vi "Main-Control Pannel.vi"() -> ()   [LabVIEW 2014]
panel:
  in  "Wifi Channel":i32=3
  out "ERROR":bool
  in  "remote IP Address":string="192.168.1.103"
  in  "UDP setup":T1={"remote IP Address"="127.0.0.0", "remote port"=54322, "local port(Tx)"=54321, "local port(Rx)"=54323}
  in  "USRP setup":T2={"Active Antenna"="RX2", "Carrier Frequency"=0.0, "IQ Rate"=0.0, "Gain"=0.0}
  in  "device names":refnum<k15>="192.168.10.2"
  in  "USRP input cluster":T3
  in  "UDP input cluster":T4
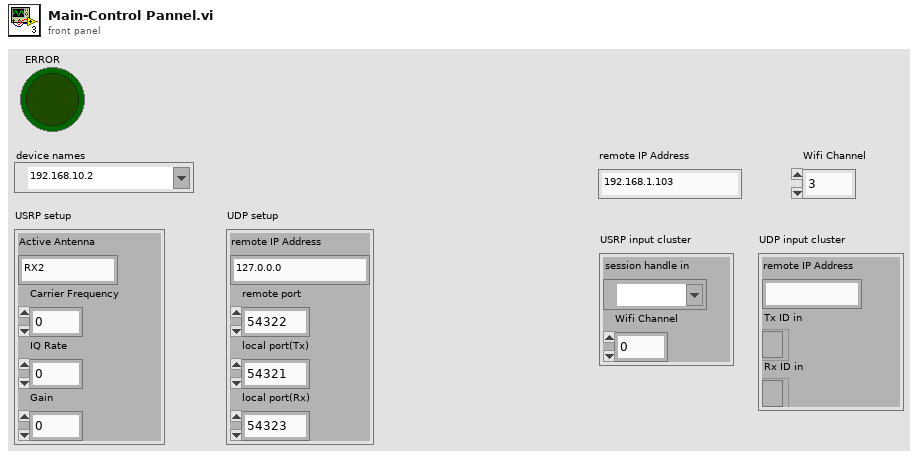
[diagram p1: front panel]
types:
  T1 = cluster{"remote IP Address":string, "remote port":u16, "local port(Tx)":u16, "local port(Rx)":u16}
  T2 = cluster{"Active Antenna":string, "Carrier Frequency":dbl, "IQ Rate":dbl, "Gain":dbl}
  T3 = cluster{"session handle in":refnum<k15>, "Wifi Channel":i32}
  T4 = cluster{"remote IP Address":string, "Tx ID in":refnum<k16>, "Rx ID in":refnum<k16>}
  T5 = cluster{"Tx ID out":refnum<k16>, "Rx ID out":refnum<k16>, "Delay Estimation":cluster{"next status(max)":i32, "next probability(max)":dbl}}
  T6 = cluster{"session handle out":refnum<k15>, "Power Estimation":cluster{"next status(max)":i32, "next probability(max)":dbl}}
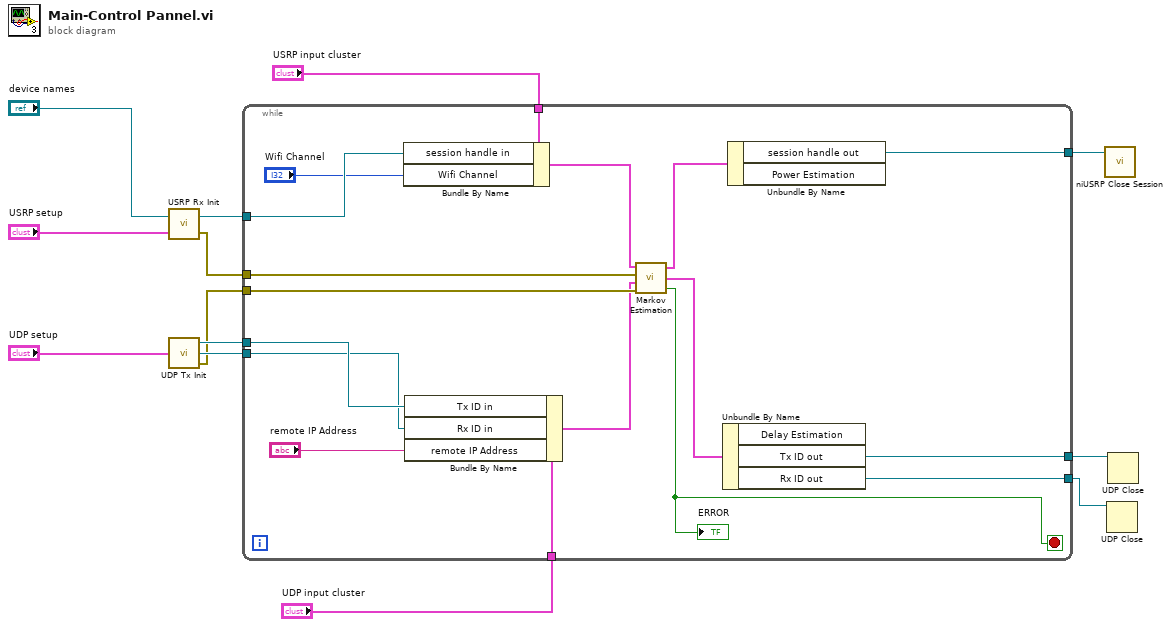
[diagram p0: block diagram]
diagram:
  n1 = call "USRP Rx Init.vi"("setup para"="USRP setup", "device names"="device names") -> ("error out"=w7:errorcluster, "session handle out"=w10:refnum<k15>)
  n2 = call "UDP Tx Init.vi"("parameter"="UDP setup") -> ("Tx ID"=w9:refnum<k16>, "Rx ID"=w8:refnum<k16>, "error out"=w6:errorcluster)  [unwired: 1 out]
  n3 = while {
    tunnel: w10 -> [w30]
    tunnel: w9 -> [w29]
    tunnel: w8 -> [w28]
    tunnel: w7 -> [w26]
    tunnel: w6 -> [w25]
    tunnel: "UDP input cluster" -> [w22]
    tunnel: "USRP input cluster" -> [w21]
    tunnel: [w18] -> w3
    tunnel: [w16] -> w2
    tunnel: [w15] -> w1
    stop <- w20 stop-if-true
    n4 = Bundle By Name(cluster=w21, "session handle in"=w30, "Wifi Channel"="Wifi Channel") -> (w23:T3)
    n5 = Bundle By Name(cluster=w22, "Tx ID in"=w29, "Rx ID in"=w28, "remote IP Address"="remote IP Address") -> (w24:T4)
    n6 = call "Markov Estimation.vi"("UDP error in"=w25, "UDP input cluster"=w24, "USRP error in"=w26, "USRP input cluster"=w23) -> ("ERROR"=w20:bool, "output cluster"=w17:T5, "USRP output cluster"=w19:T6)
    "ERROR" <- w20
    n7 = Unbundle By Name(w17) -> ("Tx ID out"=w16:refnum<k16>, "Rx ID out"=w15:refnum<k16>)  [unwired: 1 out]
    n8 = Unbundle By Name(w19) -> ("session handle out"=w18:refnum<k15>)  [unwired: 1 out]
  }
  n9 = call <instrlib>:"niUSRP Close Session.vi"("session handle"=w3) -> ()  [unwired: 14 in, 1 out]
  n10 = UDP Close(connection ID=w1) -> ()  [unwired: 1 in, 2 out]
  n11 = UDP Close(connection ID=w2) -> ()  [unwired: 1 in, 2 out]
